vi "ReadDeviceTypeAsString.vi"(8 "error in (no error)":errorcluster, 11 "GenericDevice.lvclass":refnum<class "GenericDevice.lvclass">) -> (0 "error out":errorcluster, 2 "String":string, 3 "GenericDevice.lvclass 2":refnum<class "GenericDevice.lvclass">)   [LabVIEW 2023, in "GenericDevice.lvclass"]
uses:
  GenericDevice.lvclass
  GenericDevice.lvclass/GenericDevice.ctl
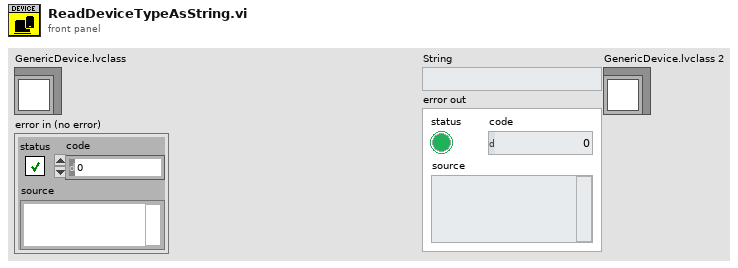
[diagram p1: front panel]
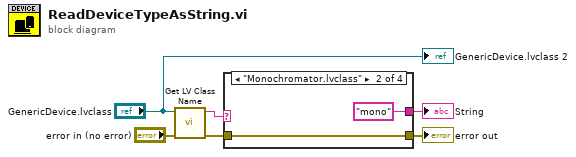
[diagram p0: block diagram]
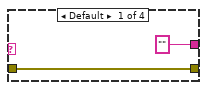
[diagram p2: hidden frame]
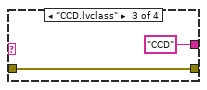
[diagram p3: hidden frame]
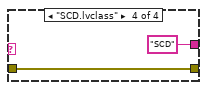
[diagram p4: hidden frame]
diagram:
  n1 = call <vilib>:"Get LV Class Name.vi"("error in (no error)"="error in (no error)", "object"="GenericDevice.lvclass") -> ("error out"=w2:errorcluster, "class name"=w6:string)  [unwired: 8 in]
  n2 = case shown="\"Monochromator.lvclass\"" w6 {
    tunnel: ["" "mono" "CCD" "SCD"] -> w3
    tunnel: w2 -> [w7 w9 w11 w13]
    tunnel: [w7 w9 w11 w13] -> w1
    frame Default {
    }
    frame "Monochromator.lvclass" {
    }
    frame "CCD.lvclass" {
    }
    frame "SCD.lvclass" {
    }
  }
  "String" <- w3
  "error out" <- w1
  "GenericDevice.lvclass 2" <- "GenericDevice.lvclass"
